vi "fgv_Send-Serial_latlogbuf.vi"(7 "cmd":enum16{"write", "read"}(ring), 8 "error in":errorcluster, 11 "latlong":cluster{"lat":dbl, "long":dbl}={"lat"=530126.7583503594, "long"=175270.68061157822} {"lat" format="%.2f"; "long" format="%.2f"}) -> (0 "error out":errorcluster, 2 "tm out":cluster{"YE":dbl, "XN":dbl}={"YE"=530126.7583503594, "XN"=175270.68061157822} {"YE" format="%.8f"; "XN" format="%.8f"}, 3 "latlong out":cluster{"lat":dbl, "long":dbl}={"lat"=530126.7583503594, "long"=175270.68061157822} {"lat" format="%.2f"; "long" format="%.2f"})   [LabVIEW 2019]
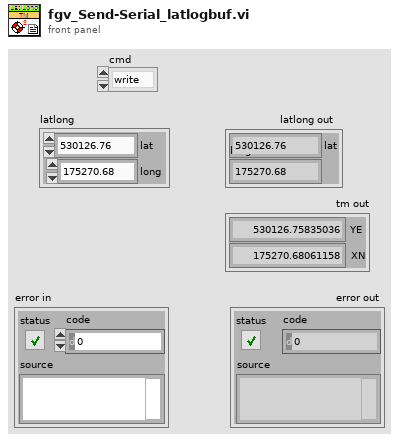
[diagram p1: front panel]
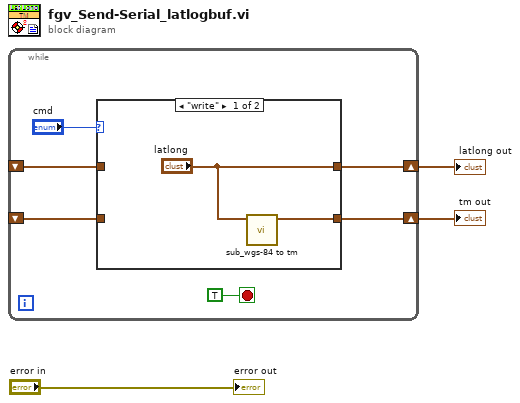
[diagram p0: block diagram]
diagram:
  n1 = while {
    shift-right: [w8] -> w3
    shift-left: _ -> [w7]
    shift-right: [w5] -> w1
    shift-left: _ -> [w4]
    stop <- TRUE stop-if-true
    n2 = case shown="\"write\"" "cmd" {
      tunnel: ["latlong" w13] -> w8
      tunnel: w7 -> [_ w13]
      tunnel: [w10 w12] -> w5
      tunnel: w4 -> [_ w12]
      frame "write" {
        n3 = call "sub_wgs-84 to tm.vi"("in_lon-lat"="latlong") -> ("TM"=w10:cluster{"Y(E)":dbl, "X(N)":dbl})  [unwired: 10 in]
      }
      frame "read", Default {
      }
    }
  }
  "latlong out" <- w3
  "tm out" <- w1
  "error out" <- "error in"
